vi "MathCad_Numeric_Get_Real.vi"(0 "Worksheet Reference In":refnum<k7>, 5 "Mathcad.INumericValue Refnum In":refnum<k7>, 11 "error in":errorcluster) -> (2 "value":dbl format="%.2f", 4 "Worksheet Reference Out":refnum<k7>, 6 "Mathcad.INumericValue Refnum Out":refnum<k7>, 15 "error out":errorcluster)   [LabVIEW 2015]
doc: "Gets the value from the reference retrieved from the getrefnum VI."
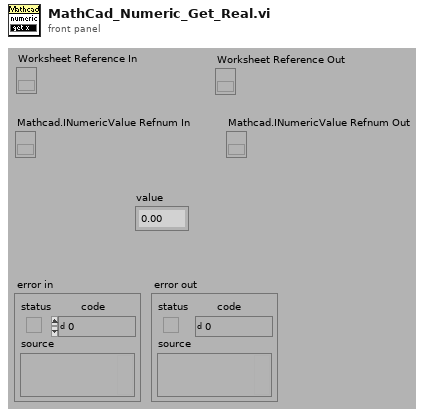
[diagram p1: front panel]
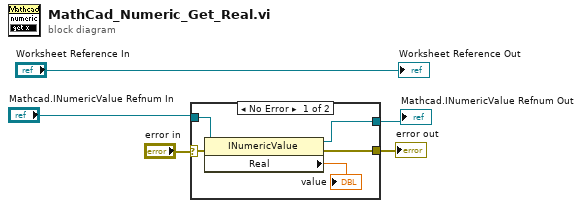
[diagram p0: block diagram]
diagram:
  n1 = case shown="No Error" "error in" {
    selector: "error in" -> [w8 w11]
    tunnel: [w6 w11] -> w5
    tunnel: "Mathcad.INumericValue Refnum In" -> [w10 w12]
    tunnel: [w7 w12] -> w2
    frame No Error {
      n2 = property class="INumericValue"(reference=w10, error in=w8) -> (reference out=w7:refnum<k7>, error out=w6:errorcluster, "Real"=→"value":dbl)
    }
    frame Error {
    }
  }
  "error out" <- w5
  "Mathcad.INumericValue Refnum Out" <- w2
  "Worksheet Reference Out" <- "Worksheet Reference In"
